vi "液位全局变量.vi"() -> ()   [LabVIEW 2010]
panel:
  out "液位增减":dbl format="%.2f"
  in  "停  止":bool
  out "容  器":dbl format="%.2f"
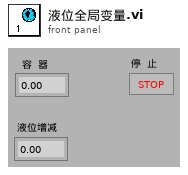
[diagram p1: front panel]
diagram:
